vi "RTDs.vi"() -> ()   [LabVIEW 2017]
uses:
  <vilib>/Platform/TimedLoop/XDataNode/timing_clust.ctl
  <vilib>/Platform/TimedLoop/XDataNode/nitl_modes.ctl
  <vilib>/Platform/TimedLoop/XDataNode/wakeup.ctl
  <vilib>/Platform/TimedLoop/XDataNode/loadnilvce.vi
  <vilib>/platform/TimedLoop/XDataNode/XDataNode.xnode
  <vilib>/Platform/TimedLoop/XDataNode/XDNodeRunTimeDep.lvlib
  <vilib>/ptbypt/NI_PtbyPt.lvlib
panel:
  in  "stop":bool
  out "RTD 2":dbl
  out "RTD 1":dbl
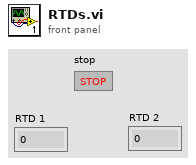
[diagram p1: front panel]
types:
  T1 = typedef "XDNodeRunTimeDep.lvlib/timing_clust.ctl" = cluster{"Expected End [f-1]":u64, "Actual End [f-1]":u64, "Finished Late? [f-1]":bool, "Expected End [i-1]":u64, "Actual End [i-1]":u64, "Finished Late? [i-1]":bool, "Expected Start [i]":u64, "Actual Start [i]":u64, "Expected Start [f]":u64, "Actual Start [f]":u64, "Source Name":string, "Structure Name":string, "Period":i64, "Deadline":i64, "Offset":i64, "Start":i64, "Priority":i32, "Timeout":i32, "Mode":T2, "Wakeup Reason":T3, "Error":errorcluster, "Source Type":string, "Secondary Source Type":string, "Global End Time":u64, "Global Start Time":u64, "Frame Duration":u64, "Iteration Duration":u64, "Assigned CPU":i32, "I/O Scan Engine Mode":u32}
  T2 = typedef "XDNodeRunTimeDep.lvlib/nitl_modes.ctl" = enum32{"No Change", "Process missed periods, maintain original phase", "Discard missed periods, maintain original phase", "Process missed periods, ignore original phase", "Discard missed periods, ignore original phase"}
  T3 = typedef "XDNodeRunTimeDep.lvlib/wakeup.ctl" = enum32{"Normal", "Aborted", "Asynchronous wakeup", "Timing source error", "Timed loop error", "Timeout"}
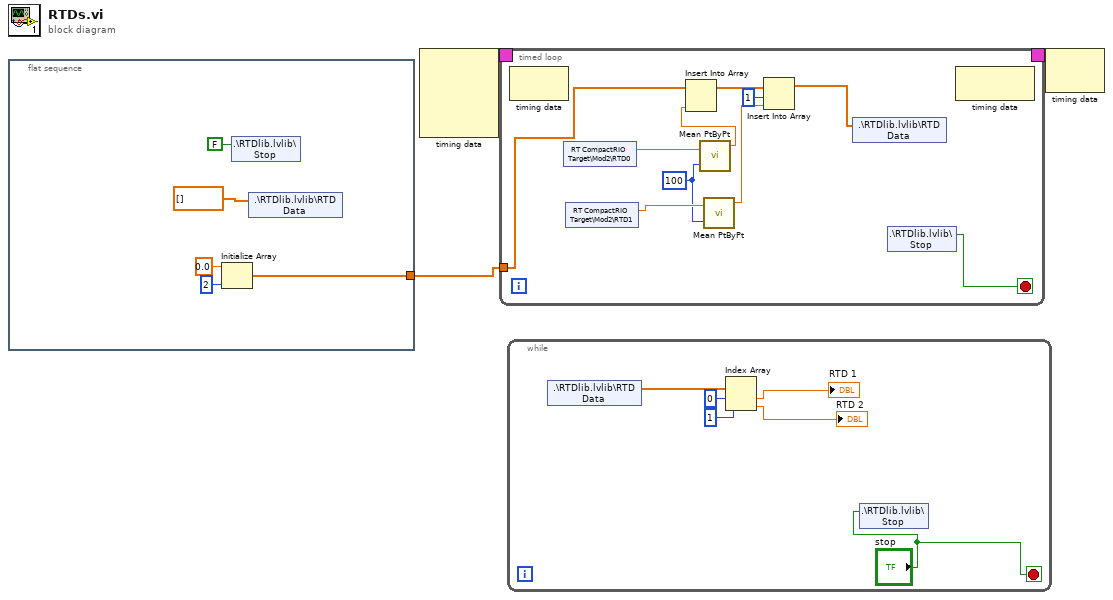
[diagram p0: block diagram]
diagram:
  n1 = flat-sequence {
    tunnel: [w4] -> w1
    frame #0 {
      n2 = Initialize Array(0.0 ("element"), 2 ("dimension size")) -> (w4:dbl[])
      n3 = shared-variable ".\\RTDlib.lvlib\\Stop"(FALSE ("Stop")) -> ()  [unwired: 1 in, 1 out]
      n4 = shared-variable ".\\RTDlib.lvlib\\RTD Data"(dbl[] [] ("RTD Data")) -> ()  [unwired: 1 in, 1 out]
    }
  }
  n5 = node-c288() -> (w3:T1)  [unwired: 4 in]
  n6 = timed-loop {
    timing: w3 -> [_]
    timing-out: [_] -> w2
    tunnel: w1 -> [w15]
    stop <- w9 stop-if-true
    w16 = 100
    n7 = node-c288() -> ()  [unwired: 1 in, 1 out]
    n8 = shared-variable "RT CompactRIO Target\\Mod2\\RTD0"() -> (w18:dbl)  [unwired: 1 in, 1 out]
    n9 = shared-variable "RT CompactRIO Target\\Mod2\\RTD1"() -> (w17:dbl)  [unwired: 1 in, 1 out]
    n10 = call <vilib>:"Mean PtByPt.vi"("x"=w18, "sample length"=w16) -> ("mean"=w13:dbl)  [unwired: 2 in, 1 out]
    n11 = Insert Into Array(array=w15, new element=w13) -> (w14:dbl[])  [unwired: 1 in]
    n12 = call <vilib>:"Mean PtByPt.vi"("x"=w17, "sample length"=w16) -> ("mean"=w12:dbl)  [unwired: 2 in, 1 out]
    n13 = Insert Into Array(array=w14, index=1, new element=w12) -> (w10:dbl[])
    n14 = shared-variable ".\\RTDlib.lvlib\\RTD Data"(w10) -> ()  [unwired: 1 in, 1 out]
    n15 = shared-variable ".\\RTDlib.lvlib\\Stop"() -> (w9:bool)  [unwired: 1 in, 1 out]
    n16 = node-c288() -> ()  [unwired: 1 in, 1 out]
  }
  n17 = while {
    stop <- "stop" stop-if-true
    n18 = shared-variable ".\\RTDlib.lvlib\\RTD Data"() -> (w26:dbl[])  [unwired: 1 in, 1 out]
    n19 = Index Array(array=w26, index #1=0 ("index"), index #2=1 ("index")) -> (element #1=→"RTD 1":dbl, element #2=→"RTD 2":dbl)
    n20 = shared-variable ".\\RTDlib.lvlib\\Stop"("stop") -> ()  [unwired: 1 in, 1 out]
  }
  n21 = node-c288(w2) -> ()  [unwired: 1 out]
